vi "GetPWD.vi"(3 "error in (no error)":errorcluster caption="错误输入（无错误）", 5 "User_Name":string) -> (0 "error out":errorcluster caption="错误输出", 1 "Permission":string, 2 "Password":string)   [LabVIEW 2020]
uses:
  <vilib>/addons/database/Connection.llb/DB Tools Open Connec (String).vi
  <vilib>/addons/database/Connection.llb/Conn Execute.vi
  <vilib>/addons/database/Recordset.llb/Rec Fetch String Data (R).vi
  <vilib>/addons/database/Recordset.llb/Rec Destroy - Connection.vi
  <vilib>/addons/database/NI_Database_API.lvlib
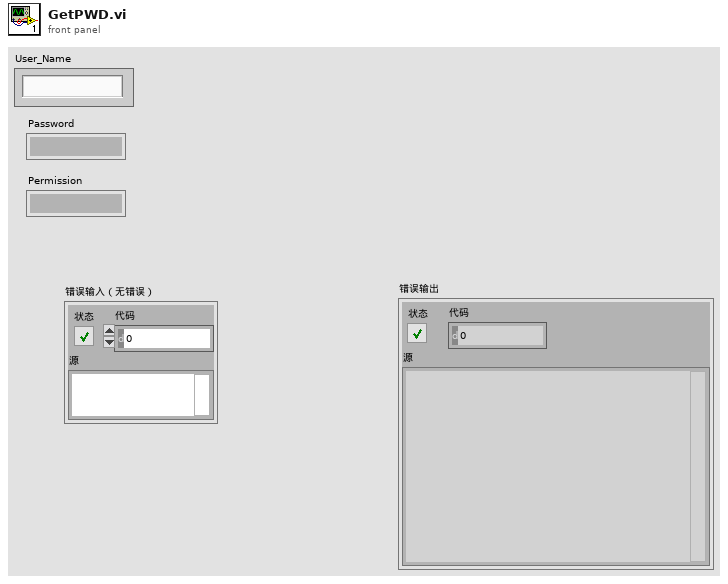
[diagram p1: front panel]
types:
  T1 = typedef "NI_Database_API.lvlib/Conn ObjectReference.ctl" = refnum<k1>
  T2 = typedef "NI_Database_API.lvlib/Rec ObjectReference.ctl" = refnum<k1>
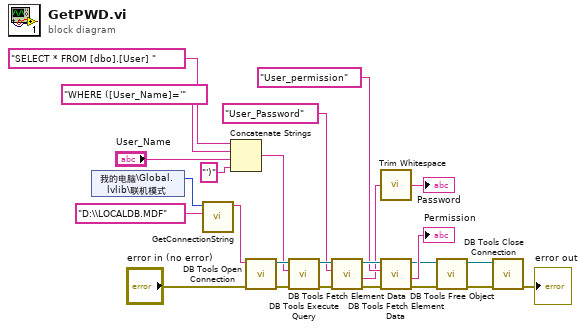
[diagram p0: block diagram]
diagram:
  n1 = shared-variable "我的电脑\\Global.lvlib\\联机模式"() -> (w4:i16)  [unwired: 1 in, 1 out]
  n2 = call "GetConnectionString.vi"("Database Name"="D:\\LOCALDB.MDF", "连接模式"=w4) -> ("连接字符串"=w5:string)  [unwired: 4 in, 1 out]
  n3 = Concatenate Strings("SELECT * FROM [dbo].[User] " ("SQL query"), "WHERE ([User_Name]='", "User_Name", "')") -> (w19:string)
  n4 = call-poly <vilib>:"DB Tools Open Connection.vi"("error in (no error)"="error in (no error)", "connection information"=w5) -> ("error out"=w17:errorcluster, "connection reference"=w25:T1)  [unwired: 6 in]
  n5 = call-poly <vilib>:"DB Tools Execute Query.vi"("error in (no error)"=w17, "SQL query"=w19, "connection reference"=w25) -> ("error out"=w16:errorcluster, "recordset reference"=w24:T2)  [unwired: 5 in]
  n6 = call-poly <vilib>:"DB Tools Fetch Element Data.vi"("error in (no error)"=w16, "column index"="User_Password", "recordset reference"=w24) -> ("error out"=w15:errorcluster, "data"=w2:string, "recordset reference out"=w18:T2)  [unwired: 4 in]
  n7 = call <vilib>:"Trim Whitespace.vi"("string"=w2) -> ("trimmed string"=→"Password":string)  [unwired: 1 in]
  n8 = call-poly <vilib>:"DB Tools Fetch Element Data.vi"("error in (no error)"=w15, "column index"="User_permission", "recordset reference"=w18) -> ("error out"=w9:errorcluster, "data"=→"Permission":string, "recordset reference out"=w11:T2)  [unwired: 4 in]
  n9 = call-poly <vilib>:"DB Tools Free Object.vi"("error in (no error)"=w9, "recordset reference"=w11) -> ("error out"=w8:errorcluster, "connection reference"=w10:T1)  [unwired: 8 in]
  n10 = call <vilib>:"DB Tools Close Connection.vi"("error in (no error)"=w8, "connection reference"=w10) -> ("error out"=→"error out":errorcluster)  [unwired: 5 in]
